vi "i2clib_open.vi"(8 "error in (no error)":errorcluster, 10 "I2C Bus":T1) -> (0 "error out":errorcluster, 3 "I2C Reference Out":i32)   [LabVIEW 2017]
uses:
  <vilib>/Rock Robotics/SystemInterfaces/i2clib/i2c_bus.ctl
  <vilib>/Utility/error.llb/Error Cluster From Error Code.vi
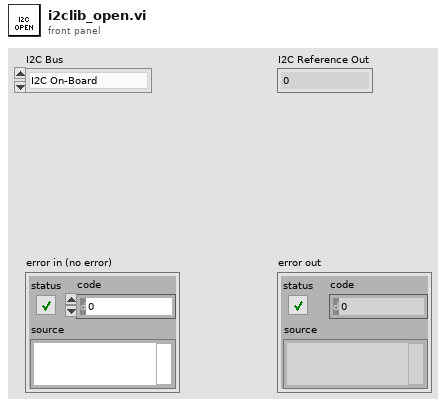
[diagram p1: front panel]
types:
  T1 = typedef "i2c_bus.ctl" = enum16{"I2C On-Board", "I2C MXP", "Invalid"}
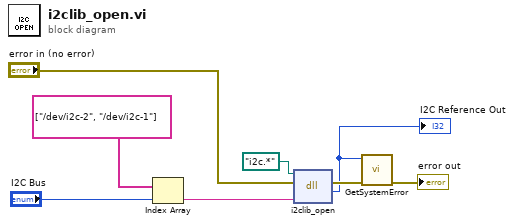
[diagram p0: block diagram]
diagram:
  n1 = Index Array(array=string[] ["/dev/i2c-2", "/dev/i2c-1"], index="I2C Bus") -> (element=w5:string)
  n2 = dll-call lib="?" fn="i2clib_open"(path in=path "i2c.*", error in="error in (no error)", "device"=w5) -> (error out=w3:errorcluster, "handle"=w1:i32)  [unwired: 2 in, 1 out]
  "I2C Reference Out" <- w1
  n3 = call <vilib>:"GetSystemError.vi"("error in (no error)"=w3, "Retval"=w1) -> ("error out"=→"error out":errorcluster)  [unwired: 9 in]
